vi "保存密码.vi"(0 "密码文件路径":path, 1 "操作人员0+密码":string[][](array[string]), 2 "管理人员1+密码":string[][](array[string])) -> (7 "错误输出":errorcluster)   [LabVIEW 2018]
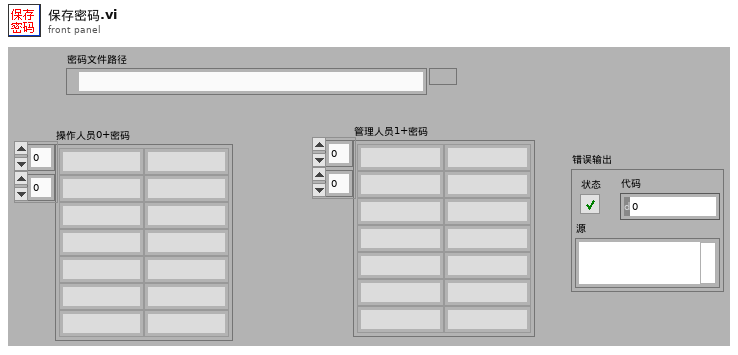
[diagram p1: front panel]
types:
  T1 = enum16{"open", "replace", "create", "open or create", "replace or create", "replace or create with confirmation"}
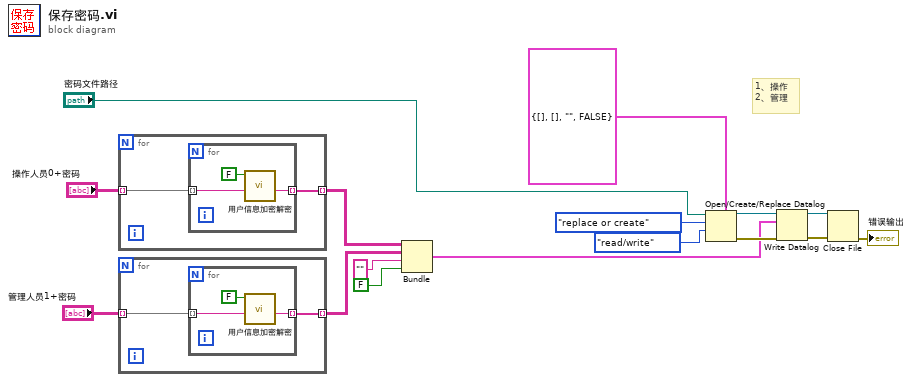
[diagram p0: block diagram]
diagram:
  # "1、操作\n2、管理"
  n1 = for {
    tunnel: "操作人员0+密码" -> [w18] mode=indexing
    tunnel: [w17] -> w16 mode=indexing
    n2 = for {
      tunnel: w18 -> [w20] mode=indexing
      tunnel: [w19] -> w17 mode=indexing
      n3 = call "用户信息加密解密.vi"("原始字符串_in"=w20, "T解密-F加密"=FALSE) -> ("加密字符串_out"=w19:string)  [unwired: 4 in, 1 out]
    }
  }
  n4 = for {
    tunnel: "管理人员1+密码" -> [w23] mode=indexing
    tunnel: [w22] -> w13 mode=indexing
    n5 = for {
      tunnel: w23 -> [w25] mode=indexing
      tunnel: [w24] -> w22 mode=indexing
      n6 = call "用户信息加密解密.vi"("原始字符串_in"=w25, "T解密-F加密"=FALSE) -> ("加密字符串_out"=w24:string)  [unwired: 4 in, 1 out]
    }
  }
  n7 = Bundle(w16, w13, "", FALSE) -> (w2:cluster{string[][], string[][], string, bool})  [unwired: 1 in]
  n8 = Open/Create/Replace Datalog(5:cluster{string[][], string[][], string, bool} {[], [], "", FALSE}, 9:enum16{"read/write", "read-only", "write-only"}."read/write" ("权限(0:read/write)"), 10:T1."replace or create" ("操作(0:open)"), 11:"密码文件路径") -> (0:w11:errorcluster, 3:w10:refnum<k1>)  [unwired: 2 in, 1 out]
  n9 = Write Datalog(4:w11, 6:w2, 7:w10) -> (0:w12:errorcluster, 3:w1:refnum<k1>)
  n10 = Close File(refnum=w1, error in=w12) -> (error out=→"错误输出":errorcluster)  [unwired: 1 out]
